vi "Main.vi"() -> ()   [LabVIEW 2012]
panel:
  out "ZTime":sgl=1000.0
  out "error out":errorcluster
  out "Waveform Chart":cluster{dbl, dbl, "HSSRPM (RPM)":sgl}(graph)={13.536735534667969, 43093.0, "HSSRPM (RPM)"=1173.7272}
  in  "stop":bool
  # "Simple FAST Simulation Demo\nPaul Fleming 1/10/13\n\nThis small program is meant to demonstrate\nthe use of FAST for Labview\n\nNote that the display of the data in the strip chart\nis for demonstration purposes only is not recommended"
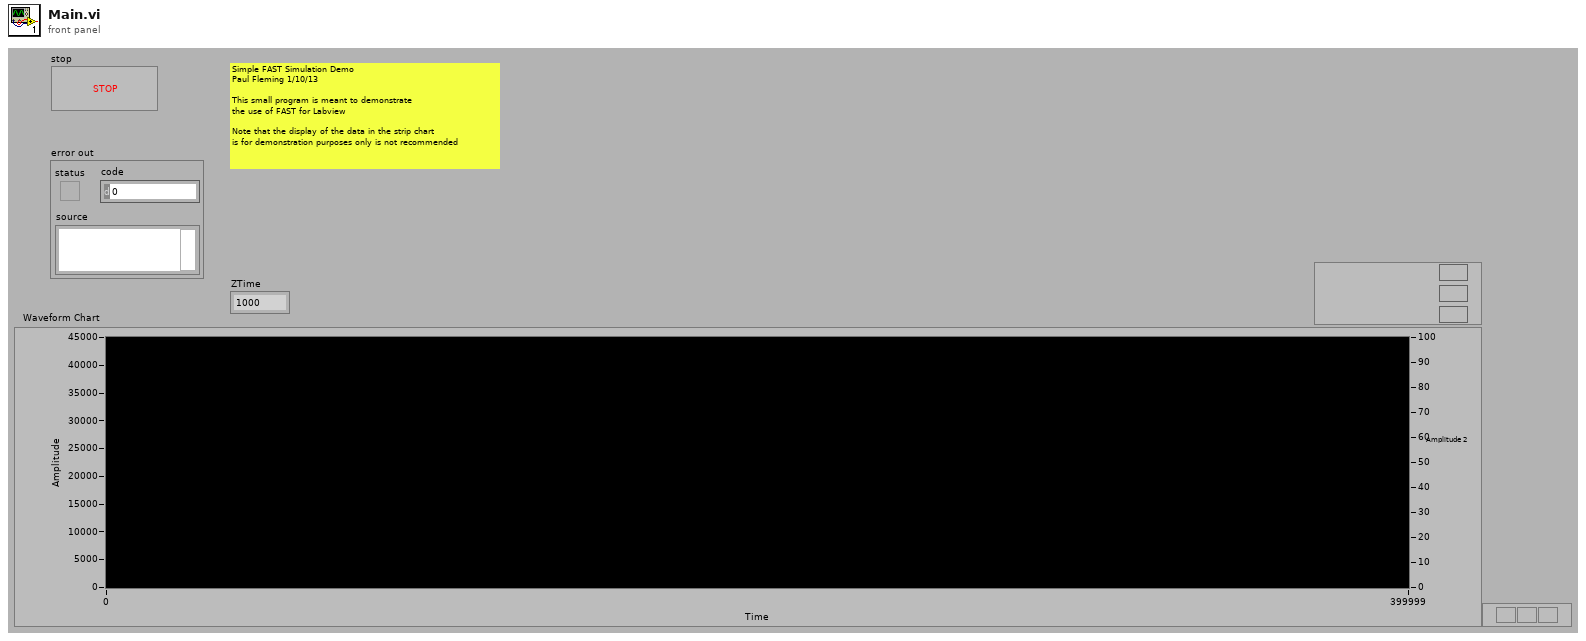
[diagram p1: front panel]
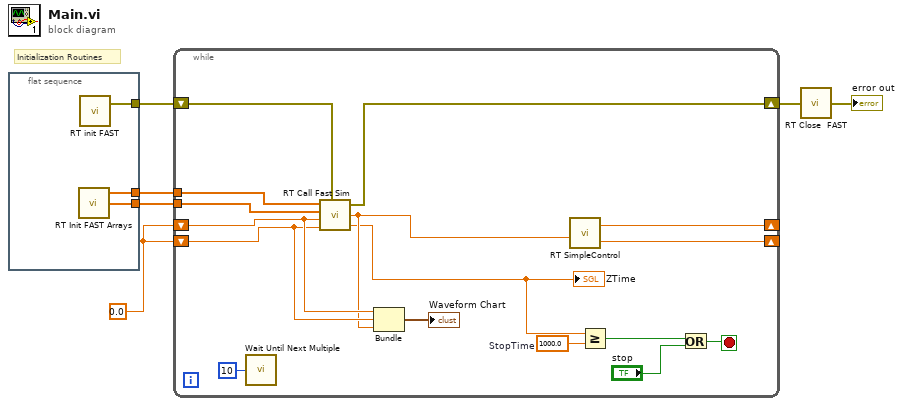
[diagram p0: block diagram]
diagram:
  w2 = 0.0
  # "Initialization Routines"
  n1 = flat-sequence {
    tunnel: [w9] -> w5
    tunnel: [w8] -> w4
    tunnel: [w7] -> w3
    frame #0 {
      n2 = call "RT Init FAST Arrays.vi"() -> ("FAST array"=w8:sgl[], "Blade Array"=w7:sgl[])  [unwired: 2 out]
      n3 = call "RT init FAST.vi"() -> ("error out"=w9:errorcluster)  [unwired: 2 out]
    }
  }
  n4 = while {
    tunnel: w4 -> [w24]
    tunnel: w3 -> [w23]
    shift-right: [w22] -> w1
    shift-left: w5 -> [w25]
    shift-right: [w21] -> _
    shift-left: w2 -> [w19]
    shift-right: [w20] -> _
    shift-left: w2 -> [w18]
    stop <- w12 stop-if-true
    w15 = sgl 1000.0  # StopTime
    n5 = call "Wait Until Next Multiple"("Count(uSec)"=u32 10) -> ()  [unwired: 1 out]
    n6 = call "RT Call Fast Sim.vi"("FAST OUT ARRAY"=w24, "BladePitchArray"=w23, "Collective Pitch Angle (Deg)"=w19, "Trq Command (Nm)"=w18, "error in (no error)"=w25) -> ("error out"=w22:errorcluster, "HSSRPM (RPM)"=w16:sgl, "ZTime"=w11:sgl)
    "ZTime" <- w11
    n7 = Bundle(w19, w18, "HSSRPM (RPM)"=w16) -> (→"Waveform Chart":cluster{dbl, dbl, "HSSRPM (RPM)":sgl})  [unwired: 1 out]
    n8 = call "RT SimpleControl.vi"("HSSRPM"=w16) -> ("Gen Torque Demand (N m)"=w20:sgl, "ColPitchDemand (Deg)"=w21:sgl)  [unwired: 9 out]
    n9 = Greater Or Equal?(x=w11, y=w15) -> (x >= y?=w14:bool)
    n10 = Or(x=w14, y="stop") -> (x .or. y?=w12:bool)
  }
  n11 = call "RT Close  FAST.vi"("error in (no error)"=w1) -> ("error out"=→"error out":errorcluster)
